vi "Final EGSA project.vi"() -> ()   [LabVIEW 2021]
panel:
  in  "stop":bool
  in  "Tab Control":T1(tab)
  in  "Password":string
  in  "User name":string
  in  "Cancel":bool
  in  "Log in":bool
  in  "Max Elevation":bool
  in  "Light&shadow":bool
  in  "Longitude":dbl
  in  "Latitude":dbl
  in  "timestep":string(combo)
  in  "end":string
  in  "Start":string
  in  "Drop your TLE path":path
  in  "Session Time":bool
  in  "Ground Track":bool
  in  "Lat & lon":bool
  in  "Log out":bool
  in  "Satellite Position":bool
  in  "Orbital Elements":bool
  out "Classification":string
  out "Epoch day of year":string
  out "Epoch year":string
  out "Launch Number of the year":string
  out "RAAN":string
  out "Inclination":string
  out "Mean anamoly":string
  out "Argument of perigee":string
  out "Eccentricty":string
  out "Piece of launch":string
  out "Line number 2":string
  out "Line number":string
  out "Satellite catalog number 2":string
  out "Satellite catalog number 1":string
  out "Last two digits of launch year":string
  in  "Menu":bool
  out "Your TLE":string
  out "Postion & Velocity":string
  out "Lat & Lon":string
  out "Boolean":bool
  out "XY Graph":cluster{"X":dbl, "Y":dbl}[](graph)
  out "String":string
  in  "Show Az & El":bool
  in  "Select your session":string(combo)
  out "Sessions":string
  out "session":string
  out "Light & Shadow":string
  # "Please enter your session in the following form : Y-M-D 00:00:00.00"
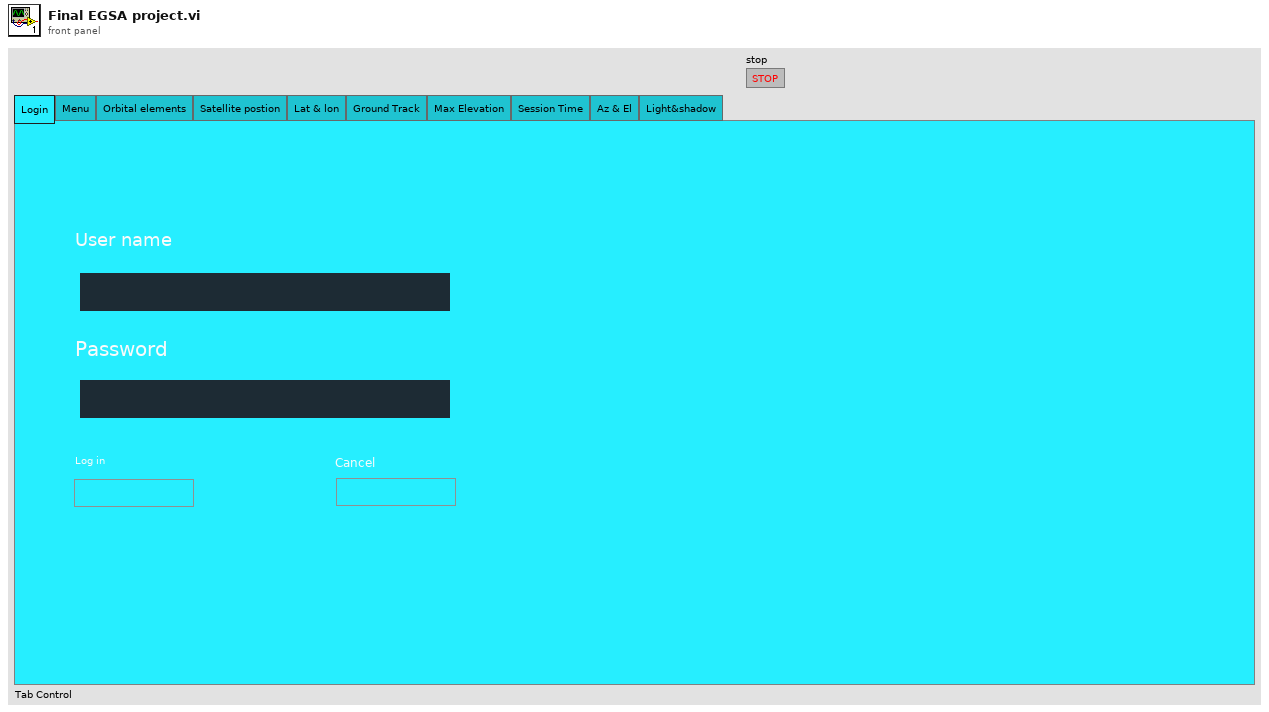
[diagram p1: front panel]
types:
  T1 = enum32{"Login", "Menu", "Orbital elements", "Satellite postion", "Lat & lon", "Ground Track", "Max Elevation", "Session Time", "Az & El", "Light&shadow"}
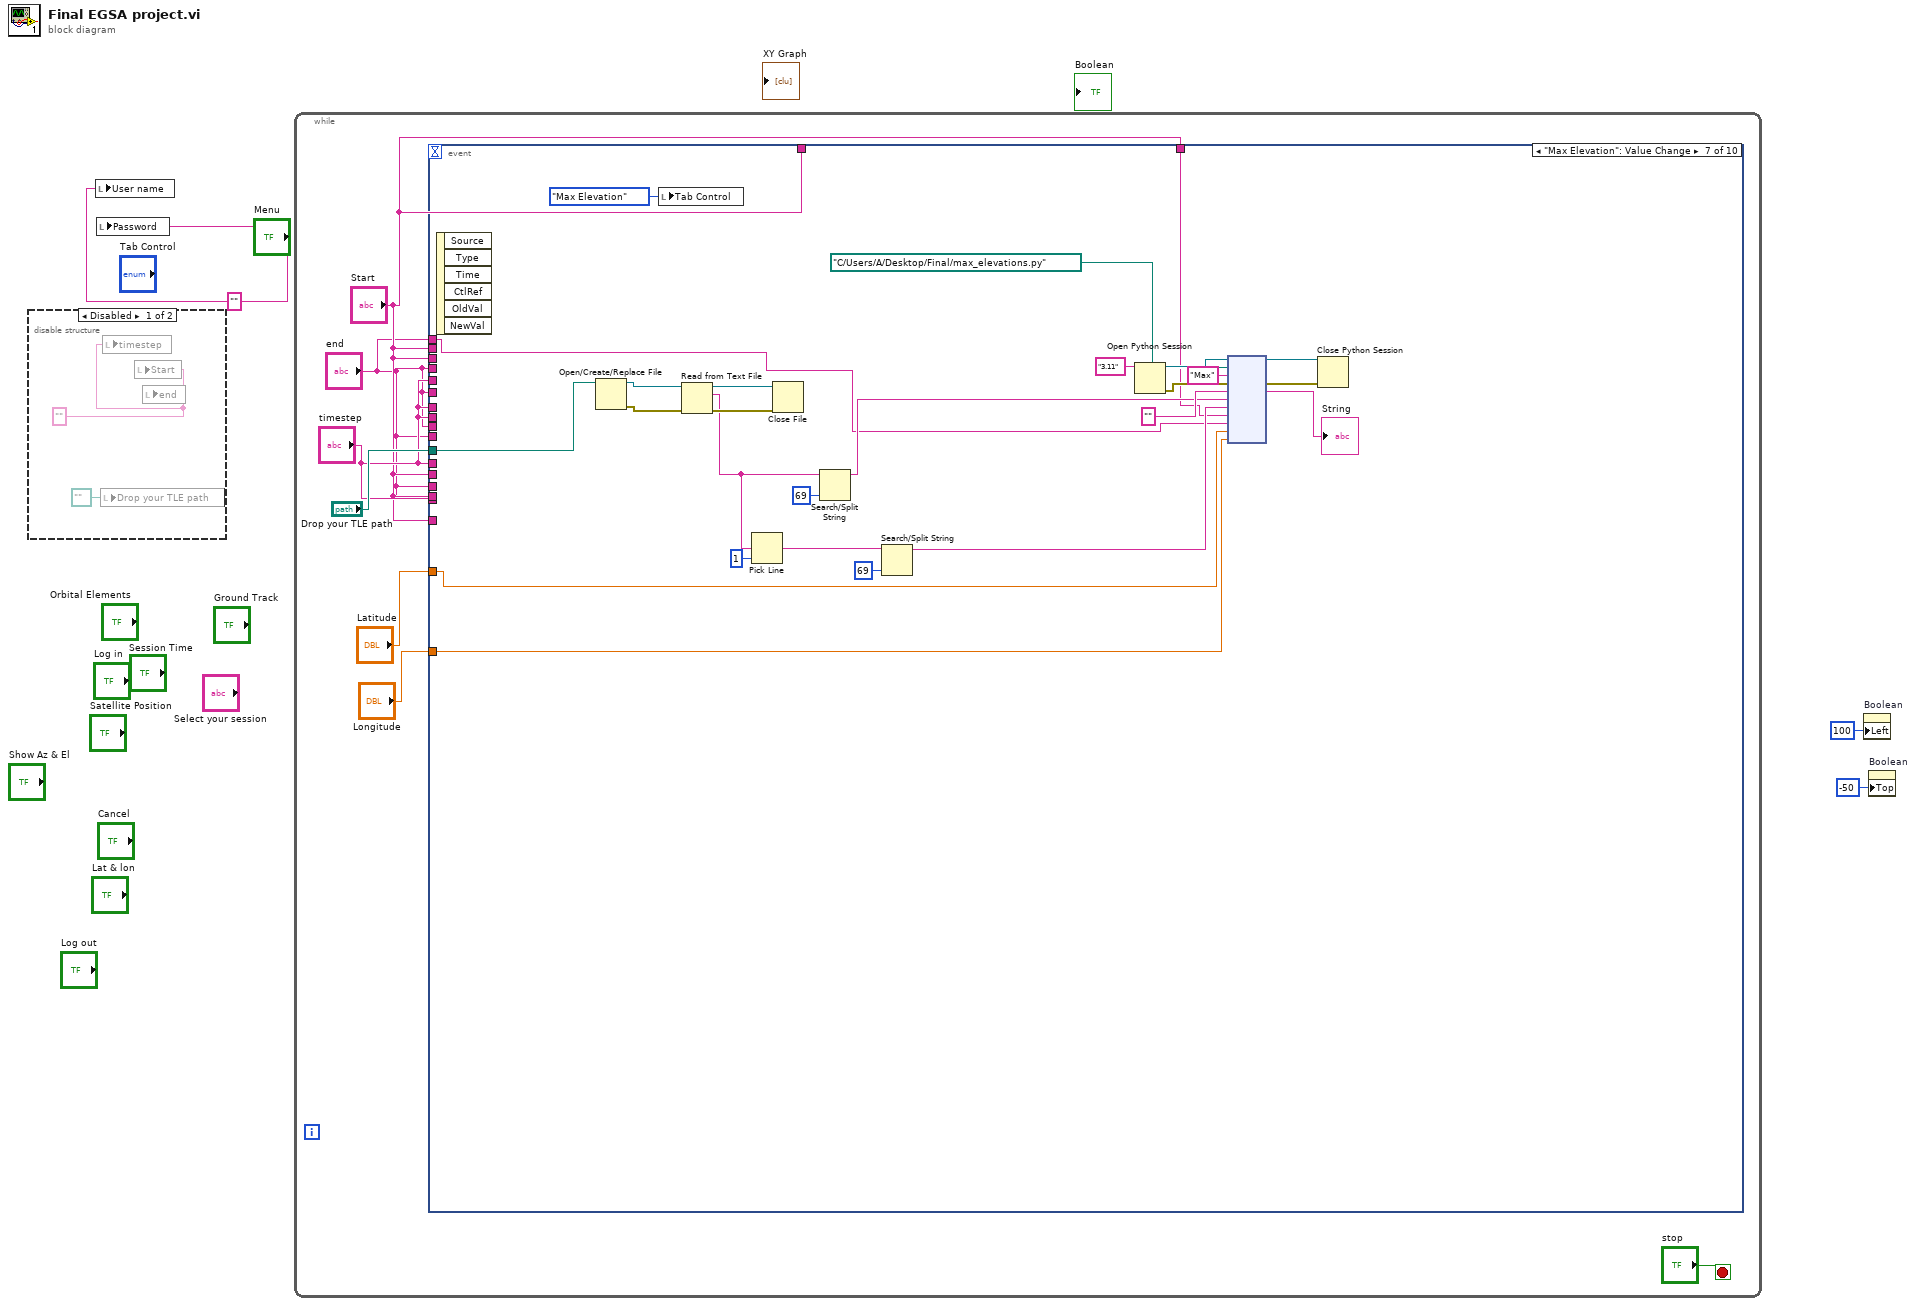
[diagram p0: block diagram]
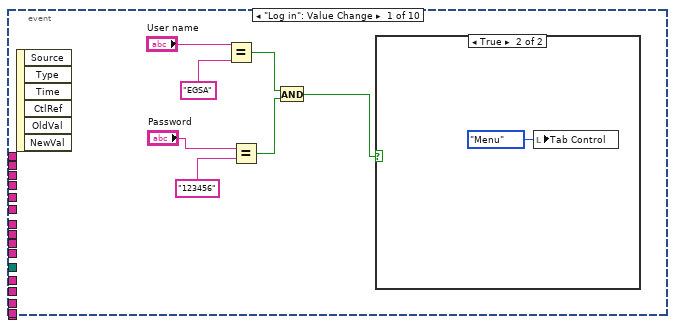
[diagram p3: hidden frame]
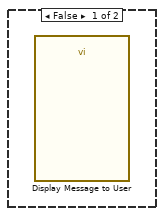
[diagram p4: hidden frame]
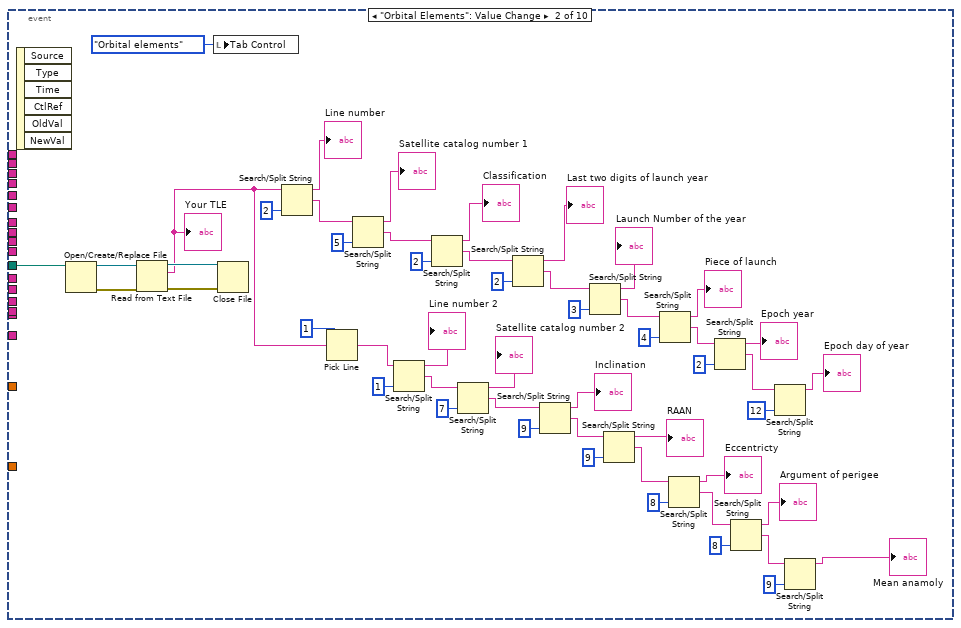
[diagram p5: hidden frame]
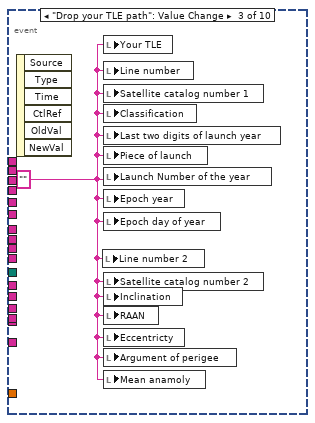
[diagram p6: hidden frame]
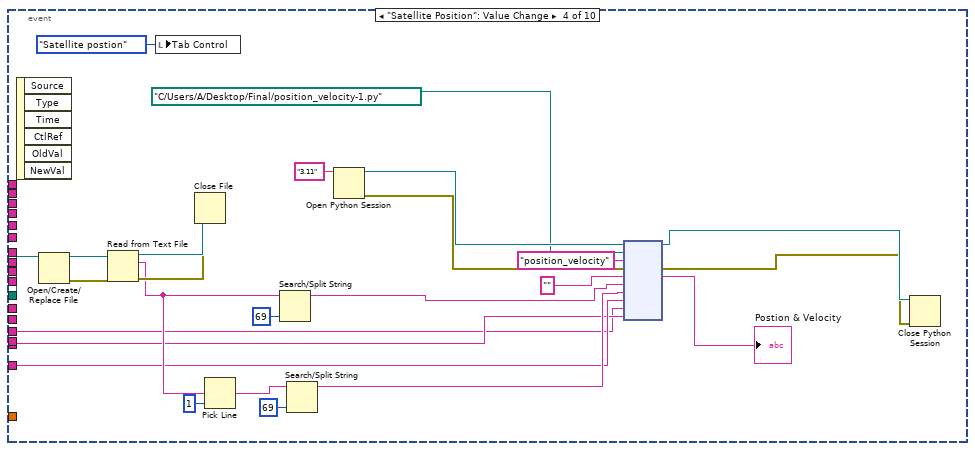
[diagram p7: hidden frame]
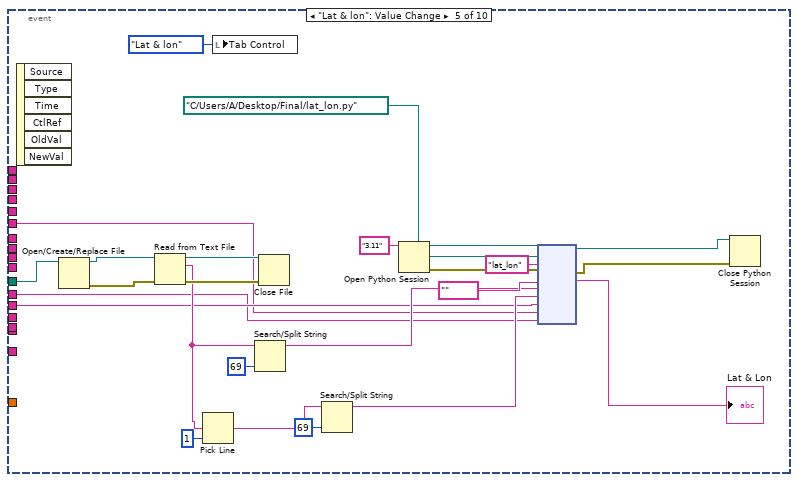
[diagram p8: hidden frame]
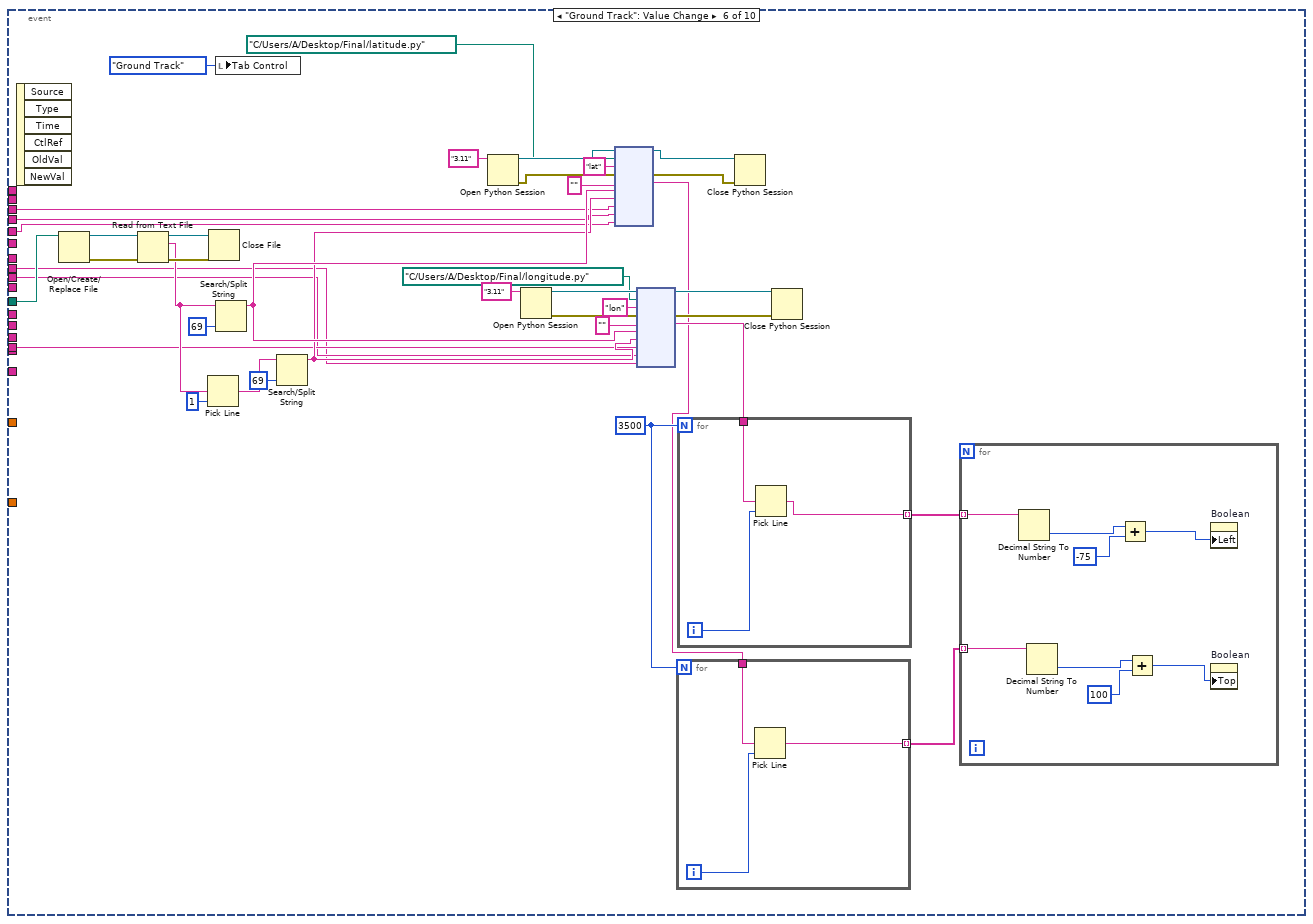
[diagram p9: hidden frame]
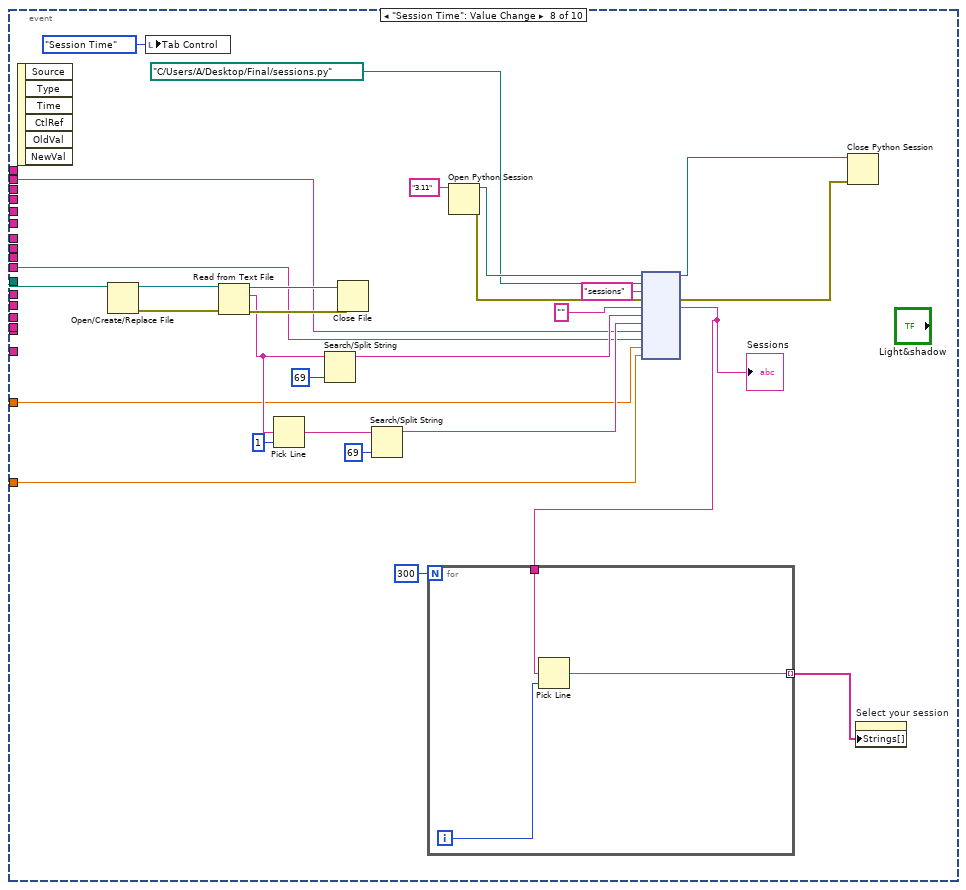
[diagram p10: hidden frame]
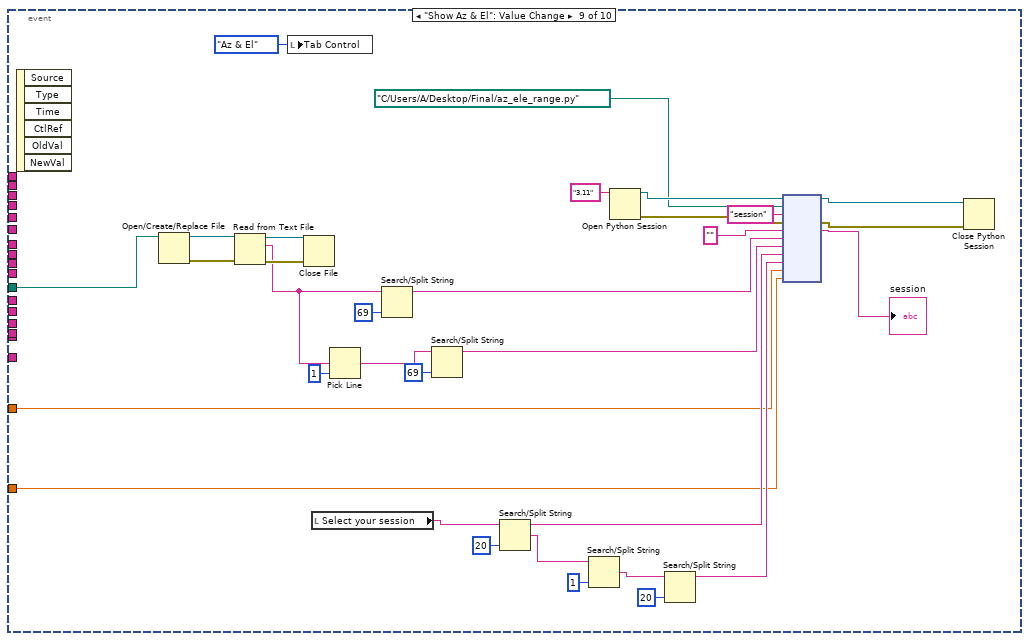
[diagram p11: hidden frame]
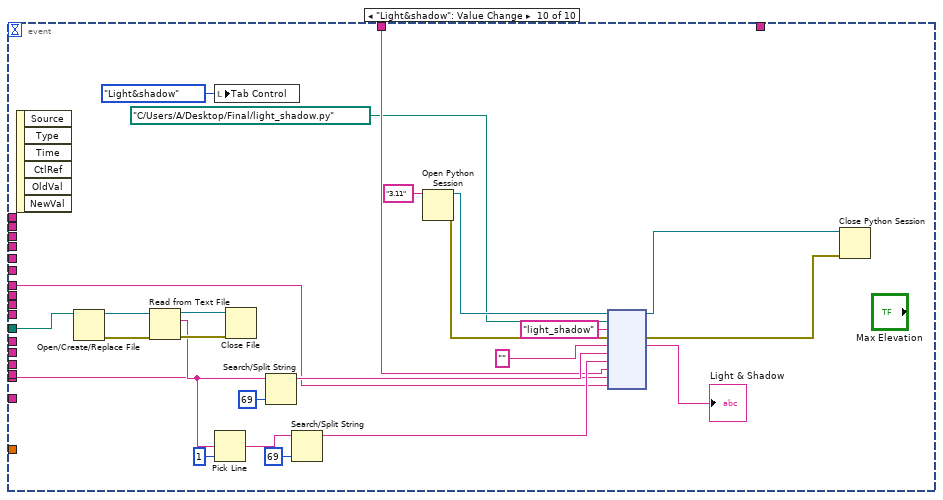
[diagram p12: hidden frame]
diagram:
  w3 = "" ("User name")
  n1 = disable-structure shown="Disabled" {
    frame Disabled {
      w5 = "" ("Start1")
      n2 = local write "Drop your TLE path"(path "" ("Drop your TLE path")) -> ()
      n3 = local write "timestep"(w5) -> ()
      n4 = local write "Start"(w5) -> ()
      n5 = local write "end"(w5) -> ()
    }
    frame Enabled {
    }
  }
  n6 = local write "User name"(w3) -> ()
  n7 = local write "Password"(w3) -> ()
  n8 = while {
    stop <- "stop" stop-if-true
    n9 = event shown="[6] \"Max Elevation\": Value Change" {
      selector: _ -> [_ _ _ _ _ _ _ _ _ _]
      dyn-events: _ -> [_ _ _ _ _ _ _ _ _ _]
      timeout: _ -> [_ _ _ _ _ _ _ _ _ _]
      tunnel: "Drop your TLE path" -> [_ w72 _ w98 w123 w143 w190 w227 w261 w287]
      tunnel: "Start" -> [_ _ _ w80 _ _ _ _ _ _]
      tunnel: "timestep" -> [_ _ _ w79 _ _ _ _ _ _]
      tunnel: "end" -> [_ _ _ w78 _ _ _ _ _ _]
      tunnel: "Start" -> [_ _ _ _ w106 _ _ _ _ _]
      tunnel: "end" -> [_ _ _ _ w105 _ _ _ _ _]
      tunnel: "timestep" -> [_ _ _ _ w104 _ _ _ _ _]
      tunnel: "Start" -> [_ _ _ _ _ _ _ w211 _ _]
      tunnel: "end" -> [_ _ _ _ _ _ _ w210 _ _]
      tunnel: "Latitude" -> [_ _ _ _ _ _ w179 w209 w237 _]
      tunnel: "Longitude" -> [_ _ _ _ _ _ w178 w208 w236 _]
      tunnel: "Start" -> [_ _ _ _ _ _ _ _ _ w274]
      tunnel: "end" -> [_ _ _ _ _ _ _ _ _ w273]
      tunnel: "timestep" -> [_ _ _ _ _ _ _ _ _ w272]
      tunnel: "Start" -> [_ _ _ _ _ w135 _ _ _ _]
      tunnel: "Start" -> [_ _ _ _ _ w134 _ _ _ _]
      tunnel: "end" -> [_ _ _ _ _ w133 _ _ _ _]
      tunnel: "end" -> [_ _ _ _ _ w132 _ _ _ _]
      tunnel: "timestep" -> [_ _ _ _ _ w131 _ _ _ _]
      tunnel: "timestep" -> [_ _ _ _ _ w130 _ _ _ _]
      tunnel: "Start" -> [_ _ _ _ _ _ w182 _ _ _]
      tunnel: "end" -> [_ _ _ _ _ _ w180 _ _ _]
      event "Log in": Value Change {
        n10 = event-data() -> ()  [unwired: 1 in, 6 out]
        n11 = Equal?(x="User name", y="EGSA") -> (x = y?=w14:bool)
        n12 = Equal?(x="Password", y="123456") -> (x = y?=w15:bool)
        n13 = And(x=w14, y=w15) -> (x .and. y?=w13:bool)
        n14 = case shown="True" w13 {
          frame False {
            n15 = call "Display Message to User"() -> ()  [unwired: 10 in, 2 out]
          }
          frame True {
            n16 = local write "Tab Control"(T1."Menu" ("Tab Control")) -> ()
          }
        }
      }
      event "Orbital Elements": Value Change {
        n17 = event-data() -> ()  [unwired: 1 in, 6 out]
        n18 = Open/Create/Replace File(file path (use dialog)=w72) -> (refnum out=w71:refnum<file>, error out=w70:errorcluster)  [unwired: 5 in, 1 out]
        n19 = Read from Text File(file (use dialog)=w71, error in=w70) -> (refnum out=w69:refnum<file>, text=w44:string, error out=w68:errorcluster)  [unwired: 2 in, 1 out]
        "Your TLE" <- w44
        n20 = local write "Tab Control"(T1."Orbital elements" ("Tab Control")) -> ()
        n21 = Close File(refnum=w69, error in=w68) -> ()  [unwired: 2 out]
        n22 = Search/Split String(string=w44, offset (0)=2) -> (substring before match=→"Line number":string, match + rest of string=w65:string)  [unwired: 1 in, 1 out]
        n23 = Pick Line(multi-line string=w44, line index=1) -> (output string=w42:string)  [unwired: 1 in]
        n24 = Search/Split String(string=w65, offset (0)=5) -> (substring before match=→"Satellite catalog number 1":string, match + rest of string=w62:string)  [unwired: 1 in, 1 out]
        n25 = Search/Split String(string=w42, offset (0)=1) -> (substring before match=→"Line number 2":string, match + rest of string=w39:string)  [unwired: 1 in, 1 out]
        n26 = Search/Split String(string=w62, offset (0)=2) -> (substring before match=→"Classification":string, match + rest of string=w59:string)  [unwired: 1 in, 1 out]
        n27 = Search/Split String(string=w39, offset (0)=7) -> (substring before match=→"Satellite catalog number 2":string, match + rest of string=w36:string)  [unwired: 1 in, 1 out]
        n28 = Search/Split String(string=w59, offset (0)=2) -> (substring before match=→"Last two digits of launch year":string, match + rest of string=w56:string)  [unwired: 1 in, 1 out]
        n29 = Search/Split String(string=w36, offset (0)=9) -> (substring before match=→"Inclination":string, match + rest of string=w33:string)  [unwired: 1 in, 1 out]
        n30 = Search/Split String(string=w56, offset (0)=3) -> (substring before match=→"Launch Number of the year":string, match + rest of string=w53:string)  [unwired: 1 in, 1 out]
        n31 = Search/Split String(string=w33, offset (0)=9) -> (substring before match=→"RAAN":string, match + rest of string=w30:string)  [unwired: 1 in, 1 out]
        n32 = Search/Split String(string=w53, offset (0)=4) -> (substring before match=→"Piece of launch":string, match + rest of string=w50:string)  [unwired: 1 in, 1 out]
        n33 = Search/Split String(string=w30, offset (0)=8) -> (substring before match=→"Eccentricty":string, match + rest of string=w27:string)  [unwired: 1 in, 1 out]
        n34 = Search/Split String(string=w50, offset (0)=2) -> (substring before match=→"Epoch year":string, match + rest of string=w47:string)  [unwired: 1 in, 1 out]
        n35 = Search/Split String(string=w27, offset (0)=8) -> (substring before match=→"Argument of perigee":string, match + rest of string=w24:string)  [unwired: 1 in, 1 out]
        n36 = Search/Split String(string=w47, offset (0)=12) -> (substring before match=→"Epoch day of year":string)  [unwired: 1 in, 2 out]
        n37 = Search/Split String(string=w24, offset (0)=9) -> (substring before match=→"Mean anamoly":string)  [unwired: 1 in, 2 out]
      }
      event "Drop your TLE path": Value Change {
        w73 = ""
        n38 = event-data() -> ()  [unwired: 1 in, 6 out]
        n39 = local write "Line number 2"(w73) -> ()
        n40 = local write "Your TLE"(w73) -> ()
        n41 = local write "Line number"(w73) -> ()
        n42 = local write "Satellite catalog number 1"(w73) -> ()
        n43 = local write "Classification"(w73) -> ()
        n44 = local write "Last two digits of launch year"(w73) -> ()
        n45 = local write "Piece of launch"(w73) -> ()
        n46 = local write "Launch Number of the year"(w73) -> ()
        n47 = local write "Epoch year"(w73) -> ()
        n48 = local write "Epoch day of year"(w73) -> ()
        n49 = local write "Satellite catalog number 2"(w73) -> ()
        n50 = local write "Inclination"(w73) -> ()
        n51 = local write "RAAN"(w73) -> ()
        n52 = local write "Eccentricty"(w73) -> ()
        n53 = local write "Argument of perigee"(w73) -> ()
        n54 = local write "Mean anamoly"(w73) -> ()
      }
      event "Satellite Position": Value Change {
        n55 = event-data() -> ()  [unwired: 1 in, 6 out]
        n56 = Open/Create/Replace File(file path (use dialog)=w98) -> (refnum out=w97:refnum<file>, error out=w96:errorcluster)  [unwired: 5 in, 1 out]
        n57 = Read from Text File(file (use dialog)=w97, error in=w96) -> (refnum out=w95:refnum<file>, text=w92:string, error out=w94:errorcluster)  [unwired: 2 in, 1 out]
        n58 = local write "Tab Control"(T1."Satellite postion" ("Tab Control")) -> ()
        n59 = Close File(refnum=w95, error in=w94) -> ()  [unwired: 2 out]
        n60 = Pick Line(multi-line string=w92, line index=1) -> (output string=w90:string)  [unwired: 1 in]
        n61 = Search/Split String(string=w92, offset (0)=69) -> (substring before match=w82:string)  [unwired: 1 in, 2 out]
        n62 = Search/Split String(string=w90, offset (0)=69) -> (substring before match=w81:string)  [unwired: 1 in, 2 out]
        n63 = Open Python Session(python version="3.11" ("Python version")) -> (session out=w88:refnum<k35>, error out=w87:errorcluster)  [unwired: 2 in]
        n64 = node(w88, path "C:/Users/A/Desktop/Final/position_velocity-1.py" ("module path"), "position_velocity" ("function name"), w87, "", w82, w81, w80, w78, w79) -> (w86:refnum<k35>, w85:errorcluster, →"Postion & Velocity":string)  [unwired: 5 in, 2 out]
        n65 = Close Python Session(session in=w86, error in=w85) -> ()  [unwired: 1 out]
      }
      event "Lat & lon": Value Change {
        n66 = event-data() -> ()  [unwired: 1 in, 6 out]
        n67 = Open/Create/Replace File(file path (use dialog)=w123) -> (refnum out=w122:refnum<file>, error out=w121:errorcluster)  [unwired: 5 in, 1 out]
        n68 = Read from Text File(file (use dialog)=w122, error in=w121) -> (refnum out=w120:refnum<file>, text=w111:string, error out=w119:errorcluster)  [unwired: 2 in, 1 out]
        n69 = Pick Line(multi-line string=w111, line index=1) -> (output string=w109:string)  [unwired: 1 in]
        n70 = local write "Tab Control"(T1."Lat & lon" ("Tab Control")) -> ()
        n71 = Search/Split String(string=w111, offset (0)=69) -> (substring before match=w112:string)  [unwired: 1 in, 2 out]
        n72 = Close File(refnum=w120, error in=w119) -> ()  [unwired: 2 out]
        n73 = Search/Split String(string=w109, offset (0)=69) -> (substring before match=w107:string)  [unwired: 1 in, 2 out]
        n74 = Open Python Session(python version="3.11" ("Python version")) -> (session out=w118:refnum<k35>, error out=w117:errorcluster)  [unwired: 2 in]
        n75 = node(w118, path "C:/Users/A/Desktop/Final/lat_lon.py" ("module path"), "lat_lon" ("function name"), w117, "", w112, w107, w106, w105, w104) -> (w116:refnum<k35>, w115:errorcluster, →"Lat & Lon":string)  [unwired: 5 in, 2 out]
        n76 = Close Python Session(session in=w116, error in=w115) -> ()  [unwired: 1 out]
      }
      event "Ground Track": Value Change {
        w129 = 3500
        n77 = event-data() -> ()  [unwired: 1 in, 6 out]
        n78 = Open/Create/Replace File(file path (use dialog)=w143) -> (refnum out=w163:refnum<file>, error out=w162:errorcluster)  [unwired: 5 in, 1 out]
        n79 = Read from Text File(file (use dialog)=w163, error in=w162) -> (refnum out=w161:refnum<file>, text=w141:string, error out=w160:errorcluster)  [unwired: 2 in, 1 out]
        n80 = Pick Line(multi-line string=w141, line index=1) -> (output string=w139:string)  [unwired: 1 in]
        n81 = Close File(refnum=w161, error in=w160) -> ()  [unwired: 2 out]
        n82 = local write "Tab Control"(T1."Ground Track" ("Tab Control")) -> ()
        n83 = Search/Split String(string=w141, offset (0)=69) -> (substring before match=w137:string)  [unwired: 1 in, 2 out]
        n84 = Search/Split String(string=w139, offset (0)=69) -> (substring before match=w136:string)  [unwired: 1 in, 2 out]
        n85 = Open Python Session(python version="3.11" ("Python version")) -> (session out=w159:refnum<k35>, error out=w158:errorcluster)  [unwired: 2 in]
        n86 = Open Python Session(python version="3.11" ("Python version")) -> (session out=w155:refnum<k35>, error out=w154:errorcluster)  [unwired: 2 in]
        n87 = node(w159, path "C:/Users/A/Desktop/Final/latitude.py" ("module path"), "lat" ("function name"), w158, "", w137, w136, w135, w133, w131) -> (w157:refnum<k35>, w156:errorcluster, w125:string)  [unwired: 5 in, 2 out]
        n88 = node(w155, path "C:/Users/A/Desktop/Final/longitude.py" ("module path"), "lon" ("function name"), w154, "", w137, w136, w134, w132, w130) -> (w153:refnum<k35>, w152:errorcluster, w126:string)  [unwired: 5 in, 2 out]
        n89 = for {
          N: w129 -> [_]
          tunnel: [w173] -> w127 mode=indexing
          tunnel: w125 -> [w172]
          i -> [w174]
          n90 = Pick Line(multi-line string=w172, line index=w174) -> (output string=w173:string)  [unwired: 1 in]
        }
        n91 = for {
          N: w129 -> [_]
          tunnel: [w176] -> w128 mode=indexing
          tunnel: w126 -> [w175]
          i -> [w177]
          n92 = Pick Line(multi-line string=w175, line index=w177) -> (output string=w176:string)  [unwired: 1 in]
        }
        n93 = Close Python Session(session in=w157, error in=w156) -> ()  [unwired: 1 out]
        n94 = Close Python Session(session in=w153, error in=w152) -> ()  [unwired: 1 out]
        n95 = for {
          tunnel: w128 -> [w171] mode=indexing
          tunnel: w127 -> [w170] mode=indexing
          n96 = Decimal String To Number(string=w171) -> (number=w168:i32)  [unwired: 2 in, 1 out]
          n97 = Decimal String To Number(string=w170) -> (number=w169:i32)  [unwired: 2 in, 1 out]
          n98 = Add(x=w168, y=-75) -> (x+y=w165:i32)
          n99 = Add(x=w169, y=100) -> (x+y=w164:i32)
          n100 = property on="Boolean" class="Bool (strict)"("Left"=w165) -> ()  [unwired: 2 in, 2 out]
          n101 = property on="Boolean" class="Bool (strict)"("Top"=w164) -> ()  [unwired: 2 in, 2 out]
        }
      }
      event "Max Elevation": Value Change {
        n102 = event-data() -> ()  [unwired: 1 in, 6 out]
        n103 = Open/Create/Replace File(file path (use dialog)=w190) -> (refnum out=w202:refnum<file>, error out=w201:errorcluster)  [unwired: 5 in, 1 out]
        n104 = local write "Tab Control"(T1."Max Elevation" ("Tab Control")) -> ()
        n105 = Read from Text File(file (use dialog)=w202, error in=w201) -> (refnum out=w200:refnum<file>, text=w187:string, error out=w199:errorcluster)  [unwired: 2 in, 1 out]
        n106 = Pick Line(multi-line string=w187, line index=1) -> (output string=w185:string)  [unwired: 1 in]
        n107 = Close File(refnum=w200, error in=w199) -> ()  [unwired: 2 out]
        n108 = Search/Split String(string=w187, offset (0)=69) -> (substring before match=w188:string)  [unwired: 1 in, 2 out]
        n109 = Search/Split String(string=w185, offset (0)=69) -> (substring before match=w183:string)  [unwired: 1 in, 2 out]
        n110 = Open Python Session(python version="3.11" ("Python version")) -> (session out=w198:refnum<k35>, error out=w197:errorcluster)  [unwired: 2 in]
        n111 = node(w198, path "C:/Users/A/Desktop/Final/max_elevations.py" ("module path"), "Max" ("function name"), w197, "", w188, w183, w182, w180, w179, w178) -> (w196:refnum<k35>, w195:errorcluster, →"String":string)  [unwired: 6 in, 2 out]
        n112 = Close Python Session(session in=w196, error in=w195) -> ()  [unwired: 1 out]
      }
      event "Session Time": Value Change {
        n113 = event-data() -> ()  [unwired: 1 in, 6 out]
        n114 = Open/Create/Replace File(file path (use dialog)=w227) -> (refnum out=w231:refnum<file>, error out=w230:errorcluster)  [unwired: 5 in, 1 out]
        n115 = local write "Tab Control"(T1."Session Time" ("Tab Control")) -> ()
        n116 = Read from Text File(file (use dialog)=w231, error in=w230) -> (refnum out=w229:refnum<file>, text=w225:string, error out=w228:errorcluster)  [unwired: 2 in, 1 out]
        n117 = Pick Line(multi-line string=w225, line index=1) -> (output string=w223:string)  [unwired: 1 in]
        n118 = Search/Split String(string=w225, offset (0)=69) -> (substring before match=w213:string)  [unwired: 1 in, 2 out]
        n119 = Close File(refnum=w229, error in=w228) -> ()  [unwired: 2 out]
        n120 = Search/Split String(string=w223, offset (0)=69) -> (substring before match=w212:string)  [unwired: 1 in, 2 out]
        n121 = Open Python Session(python version="3.11" ("Python version")) -> (session out=w221:refnum<k35>, error out=w220:errorcluster)  [unwired: 2 in]
        n122 = node(w221, path "C:/Users/A/Desktop/Final/sessions.py" ("module path"), "sessions" ("function name"), w220, "", w213, w212, w211, w210, w209, w208) -> (w219:refnum<k35>, w218:errorcluster, w206:string)  [unwired: 6 in, 2 out]
        "Sessions" <- w206
        n123 = for {
          N: 300 -> [_]
          tunnel: w206 -> [w234]
          tunnel: [w232] -> w205 mode=indexing
          i -> [w233]
          n124 = Pick Line(multi-line string=w234, line index=w233) -> (output string=w232:string)  [unwired: 1 in]
        }
        n125 = Close Python Session(session in=w219, error in=w218) -> ()  [unwired: 1 out]
        n126 = property on="Select your session" class="CmbBox"("Strings[]"=w205) -> ()  [unwired: 2 in, 2 out]
      }
      event "Show Az & El": Value Change {
        n127 = event-data() -> ()  [unwired: 1 in, 6 out]
        n128 = Open/Create/Replace File(file path (use dialog)=w261) -> (refnum out=w265:refnum<file>, error out=w264:errorcluster)  [unwired: 5 in, 1 out]
        n129 = Read from Text File(file (use dialog)=w265, error in=w264) -> (refnum out=w263:refnum<file>, text=w250:string, error out=w262:errorcluster)  [unwired: 2 in, 1 out]
        n130 = local write "Tab Control"(T1."Az & El" ("Tab Control")) -> ()
        n131 = Close File(refnum=w263, error in=w262) -> ()  [unwired: 2 out]
        n132 = local read "Select your session"() -> (w245:string)
        n133 = Pick Line(multi-line string=w250, line index=1) -> (output string=w248:string)  [unwired: 1 in]
        n134 = Search/Split String(string=w250, offset (0)=69) -> (substring before match=w251:string)  [unwired: 1 in, 2 out]
        n135 = Search/Split String(string=w248, offset (0)=69) -> (substring before match=w246:string)  [unwired: 1 in, 2 out]
        n136 = Search/Split String(string=w245, offset (0)=20) -> (substring before match=w241:string, match + rest of string=w243:string)  [unwired: 1 in, 1 out]
        n137 = Search/Split String(string=w243, offset (0)=1) -> (match + rest of string=w240:string)  [unwired: 1 in, 2 out]
        n138 = Open Python Session(python version="3.11" ("Python version")) -> (session out=w260:refnum<k35>, error out=w259:errorcluster)  [unwired: 2 in]
        n139 = Search/Split String(string=w240, offset (0)=20) -> (substring before match=w238:string)  [unwired: 1 in, 2 out]
        n140 = node(w260, path "C:/Users/A/Desktop/Final/az_ele_range.py" ("module path"), "session" ("function name"), w259, "", w251, w246, w241, w238, w237, w236) -> (w258:refnum<k35>, w257:errorcluster, →"session":string)  [unwired: 6 in, 2 out]
        n141 = Close Python Session(session in=w258, error in=w257) -> ()  [unwired: 1 out]
      }
      event "Light&shadow": Value Change {
        n142 = event-data() -> ()  [unwired: 1 in, 6 out]
        n143 = Open/Create/Replace File(file path (use dialog)=w287) -> (refnum out=w291:refnum<file>, error out=w290:errorcluster)  [unwired: 5 in, 1 out]
        n144 = Read from Text File(file (use dialog)=w291, error in=w290) -> (refnum out=w289:refnum<file>, text=w281:string, error out=w288:errorcluster)  [unwired: 2 in, 1 out]
        n145 = local write "Tab Control"(T1."Light&shadow" ("Tab Control")) -> ()
        n146 = Pick Line(multi-line string=w281, line index=1) -> (output string=w279:string)  [unwired: 1 in]
        n147 = Close File(refnum=w289, error in=w288) -> ()  [unwired: 2 out]
        n148 = Search/Split String(string=w281, offset (0)=69) -> (substring before match=w276:string)  [unwired: 1 in, 2 out]
        n149 = Search/Split String(string=w279, offset (0)=69) -> (substring before match=w275:string)  [unwired: 1 in, 2 out]
        n150 = Open Python Session(python version="3.11" ("Python version")) -> (session out=w286:refnum<k35>, error out=w285:errorcluster)  [unwired: 2 in]
        n151 = node(w286, path "C:/Users/A/Desktop/Final/light_shadow.py" ("module path"), "light_shadow" ("function name"), w285, "", w276, w275, w274, w273, w272) -> (w284:refnum<k35>, w283:errorcluster, →"Light & Shadow":string)  [unwired: 5 in, 2 out]
        n152 = Close Python Session(session in=w284, error in=w283) -> ()  [unwired: 1 out]
      }
    }
  }
  n153 = property on="Boolean" class="Bool (strict)"("Left"=100 ("Position:Left")) -> ()  [unwired: 2 in, 2 out]
  n154 = property on="Boolean" class="Bool (strict)"("Top"=-50 ("Position:Top")) -> ()  [unwired: 2 in, 2 out]
